vi "util_change_in_write.vi"(8 "error in (no error)":errorcluster, 11 "data":variant) -> (0 "error out":errorcluster)   [LabVIEW 2015, in "lv-recipe-machine.lvlib"]
doc: "util_change_in_write.vi will notify the internal processes of recipe_machine that a change has occured using events, although data is not currently used, it's available to any process registered to the event."
uses:
  lv-recipe-machine.lvlib
  _controls/change.ctl
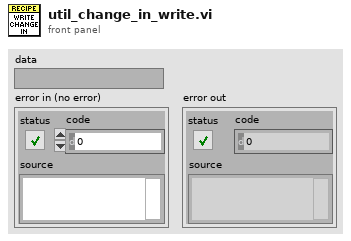
[diagram p1: front panel]
types:
  T1 = typedef "lv-recipe-machine.lvlib/change.ctl" = cluster{"data":variant}
  T2 = typedef "lv-recipe-machine.lvlib/references.ctl" = cluster{"semaphore":T3, "input_queue":refnum<queue>, "output_queue":refnum<queue>, "transition_queue":refnum<queue>, "data_dvr":refnum<data-value>, "stop_notifier":refnum<notifier>, "change_in_event":refnum<user-event>, "change_out_event":refnum<user-event>, "status_event":refnum<user-event>}
  T3 = typedef "Semaphore RefNum" = refnum<k1>
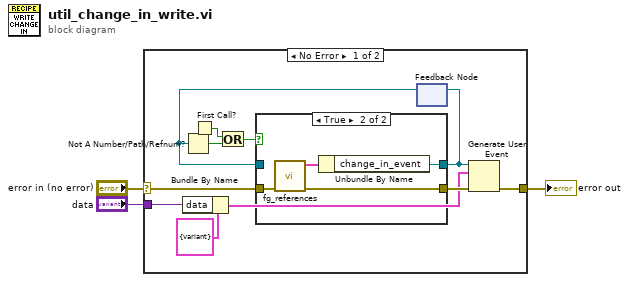
[diagram p0: block diagram]
diagram:
  n1 = case shown="No Error" "error in (no error)" {
    selector: "error in (no error)" -> [w4 w21]
    tunnel: [w13 w21] -> w3
    tunnel: "data" -> [w12 _]
    frame No Error {
      n2 = Bundle By Name(cluster=T1 {"data"=variant} ("change"), "data"=w12) -> (w10:T1)
      n3 = First Call?() -> (First Call?: T/F=w8:bool)
      n4 = feedback #1() -> (w7:refnum<user-event>)  [unwired: 1 in]
      n5 = Not A Number/Path/Refnum?(number/path/refnum=w7) -> (NaN/Path/Refnum?=w9:bool)
      n6 = Or(x=w8, y=w9) -> (x .or. y?=w6:bool)
      n7 = case shown="True" w6 {
        tunnel: w4 -> [w15 w20]
        tunnel: [w15 w19] -> w14
        tunnel: [w16 w17] -> w5
        tunnel: w7 -> [w16 _]
        frame False {
        }
        frame True {
          n8 = call "fg_references.vi"("error in (no error)"=w20) -> ("error out"=w19:errorcluster, "references out"=w18:T2)  [unwired: 9 in]
          n9 = Unbundle By Name(w18) -> ("change_in_event"=w17:refnum<user-event>)
        }
      }
      n10 = feedback-in #1(w5) -> ()
      n11 = Generate User Event(user event=w5, event data cluster=w10, error in=w14) -> (error out=w13:errorcluster)  [unwired: 1 in, 1 out]
    }
    frame Error {
    }
  }
  "error out" <- w3
